vi "reversing_feature.vi"(8 "speed in":dbl, 9 "offset angle":dbl, 10 "meas angle in":dbl, 11 "set angle in":dbl) -> (0 "speed out":dbl, 3 "set angle out":dbl)   [LabVIEW 2023]
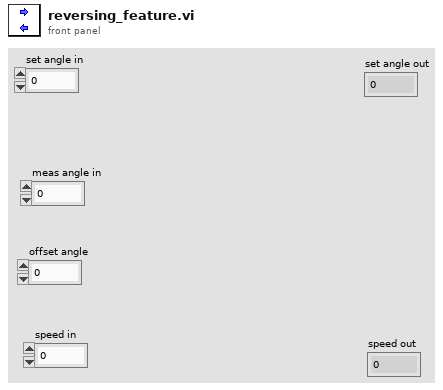
[diagram p1: front panel]
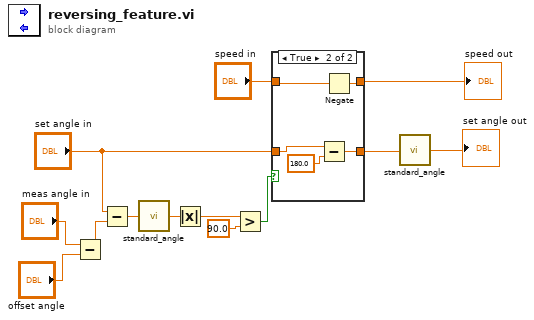
[diagram p0: block diagram]
diagram:
  n1 = Subtract(x="meas angle in", y="offset angle") -> (x-y=w2:dbl)
  n2 = Subtract(x="set angle in", y=w2) -> (x-y=w13:dbl)
  n3 = call "standard_angle.vi"("angle in"=w13) -> ("angle out"=w12:dbl)
  n4 = Absolute Value(x=w12) -> (abs(x)=w11:dbl)
  n5 = Greater?(x=w11, y=90.0) -> (0:w1:bool)
  n6 = case shown="True" w1 {
    tunnel: "set angle in" -> [w15 w16]
    tunnel: [w15 w18] -> w5
    tunnel: "speed in" -> [w14 w19]
    tunnel: [w14 w20] -> w7
    frame False {
    }
    frame True {
      n7 = Subtract(x=w16, y=180.0) -> (x-y=w18:dbl)
      n8 = Negate(x=w19) -> (-x=w20:dbl)
    }
  }
  "speed out" <- w7
  n9 = call "standard_angle.vi"("angle in"=w5) -> ("angle out"=→"set angle out":dbl)
